vi "Overlay Line with Arrows Simple Modified.vi"(0 "Image In":T2, 1 "Group":string, 2 "Angle Coefficient":dbl, 5 "Line Coordinates":T1, 9 "Arrows":cluster{"Start point":bool, "End point":bool}, 11 "error in":errorcluster, 12 "Color":u32(colorbox)=16711680, 13 "Height Coefficient":dbl) -> (4 "Image Out":T2, 15 "error out":errorcluster)   [LabVIEW 2019]
uses:
  <vilib>/vision/Image Controls.llb/IMAQ Image.ctl
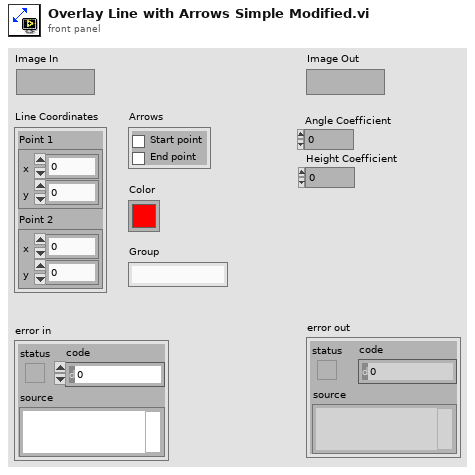
[diagram p1: front panel]
types:
  T1 = cluster{"Point 1":cluster{"x":dbl, "y":dbl}, "Point 2":cluster{"x":dbl, "y":dbl}}
  T2 = typedef "IMAQ Image.ctl" = refnum<image>
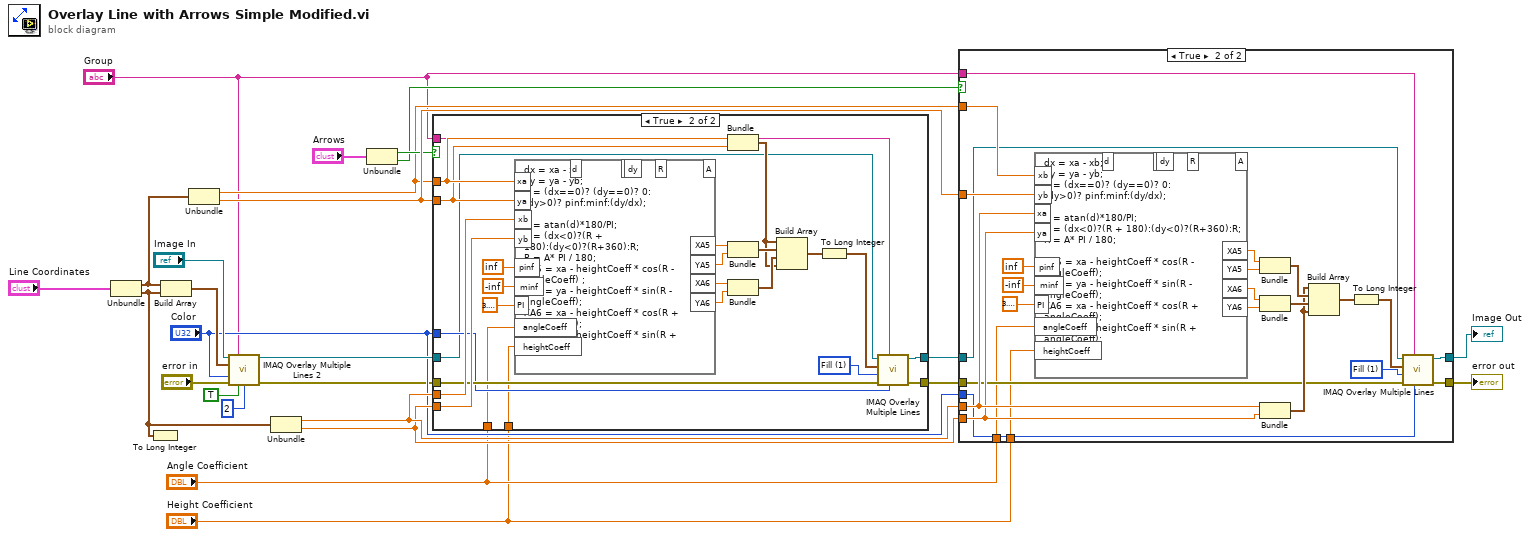
[diagram p0: block diagram]
diagram:
  n1 = Unbundle("Line Coordinates") -> ("Point 1"=w11:cluster{"x":dbl, "y":dbl}, "Point 2"=w10:cluster{"x":dbl, "y":dbl})
  n2 = To Long Integer(number=w10) -> ()  [unwired: 1 out]
  n3 = Build Array(w11, w10) -> (w9:cluster{"x":dbl, "y":dbl}[])
  n4 = Unbundle(w11) -> ("x"=w19:dbl, "y"=w24:dbl)
  n5 = call "IMAQ Overlay Multiple Lines 2"("Image"="Image In", "Group"="Group", "Line End Points"=w9, "Color"="Color", "error in (no error)"="error in", "Maintain Width?"=TRUE, "Width"=u32 2) -> ("Image Out"=w12:T2, "error out"=w6:errorcluster)  [unwired: 7 in]
  n6 = Unbundle(w10) -> ("x"=w23:dbl, "y"=w18:dbl)
  n7 = Unbundle("Arrows") -> ("Start point"=w22:bool, "End point"=w14:bool)
  n8 = case shown="True" w22 {
    tunnel: w19 -> [_ w41]
    tunnel: w24 -> [_ w40]
    tunnel: w23 -> [_ w42]
    tunnel: w18 -> [_ w39]
    tunnel: w12 -> [w27 w31]
    tunnel: [w27 w35] -> w20
    tunnel: "Color" -> [_ w32]
    tunnel: w6 -> [w26 w37]
    tunnel: [w26 w36] -> w17
    tunnel: "Group" -> [_ w30]
    tunnel: "Angle Coefficient" -> [_ w29]
    tunnel: "Height Coefficient" -> [_ w28]
    frame False {
    }
    frame True {
      w33 = u32 1 items=["Frame", "Fill"] ("Drawing Mode (Frame)")
      n9 = formula code="dx = xa - xb;\ndy = ya - yb;\nd = (dx==0)? (dy==0)? 0: \n(dy>0)? pinf:minf:(dy/dx);\n\nR = atan(d)*180/PI;\nA = (dx<0)?(R + 180):(dy<0)?(R+360):R;\nR = A* PI / 180;\nXA5 = xa - heightCoeff * cos(R - angleCoeff) ;\nYA5 = ya - heightCoeff * sin(R - angleCoeff);\nXA6 = xa - heightCoeff * cos(R + angleCoeff);\nYA6 = ya - heightCoeff * sin(R + angleCoeff);"("xa"=w41, "ya"=w40, "xb"=w42, "yb"=w39, "pinf"=inf, "minf"=-inf, "PI"=3.141592653589793, "angleCoeff"=w29, "heightCoeff"=w28) -> ("XA5"=w49:dbl, "YA5"=w48:dbl, "XA6"=w47:dbl, "YA6"=w46:dbl)  [unwired: 5 out]
      n10 = Bundle("x"=w41, "y"=w40) -> (w43:cluster{"x":dbl, "y":dbl})  [unwired: 1 out]
      n11 = Bundle("XA5"=w49, "YA5"=w48) -> (w45:cluster{"XA5":dbl, "YA5":dbl})  [unwired: 1 out]
      n12 = Bundle("XA6"=w47, "YA6"=w46) -> (w44:cluster{"XA6":dbl, "YA6":dbl})  [unwired: 1 out]
      n13 = Build Array(w43, w45, w44, w43) -> (w38:cluster{"x":dbl, "y":dbl}[])
      n14 = To Long Integer(number=w38) -> (32bit integer=w34:cluster{"x":i32, "y":i32}[])
      n15 = call "IMAQ Overlay Multiple Lines"("Color"=w32, "Group"=w30, "error in (no error)"=w37, "Drawing Mode (Frame)"=w33, "Line End Points"=w34, "Image"=w31) -> ("error out"=w36:errorcluster, "Image Out"=w35:T2)  [unwired: 4 out]
    }
  }
  n16 = case shown="True" w14 {
    tunnel: w19 -> [_ w76]
    tunnel: w24 -> [_ w75]
    tunnel: w23 -> [_ w74]
    tunnel: w18 -> [_ w73]
    tunnel: w20 -> [w54 w64]
    tunnel: [w54 w63] -> w21
    tunnel: "Color" -> [_ w59]
    tunnel: w17 -> [w53 w62]
    tunnel: [w53 w61] -> w16
    tunnel: "Group" -> [_ w57]
    tunnel: "Angle Coefficient" -> [_ w56]
    tunnel: "Height Coefficient" -> [_ w55]
    frame False {
    }
    frame True {
      w58 = u32 1 items=["Frame", "Fill"] ("Drawing Mode (Frame)")
      n17 = formula code="dx = xa - xb;\ndy = ya - yb;\nd = (dx==0)? (dy==0)? 0:\n(dy>0)? pinf:minf:(dy/dx);\n\nR = atan(d)*180/PI;\nA = (dx<0)?(R + 180):(dy<0)?(R+360):R;\nR = A* PI / 180;\n\nXA5 = xa - heightCoeff * cos(R - angleCoeff);\nYA5 = ya - heightCoeff * sin(R - angleCoeff);\nXA6 = xa - heightCoeff * cos(R + angleCoeff);\nYA6 = ya - heightCoeff * sin(R + angleCoeff);"("xb"=w76, "yb"=w75, "xa"=w74, "ya"=w73, "pinf"=inf, "minf"=-inf, "PI"=3.141592653589793, "angleCoeff"=w56, "heightCoeff"=w55) -> ("XA5"=w72:dbl, "YA5"=w71:dbl, "XA6"=w70:dbl, "YA6"=w69:dbl)  [unwired: 5 out]
      n18 = Bundle("XA5"=w72, "YA5"=w71) -> (w68:cluster{"XA5":dbl, "YA5":dbl})  [unwired: 1 out]
      n19 = Bundle("XA6"=w70, "YA6"=w69) -> (w67:cluster{"XA6":dbl, "YA6":dbl})  [unwired: 1 out]
      n20 = Bundle("x"=w74, "y"=w73) -> (w66:cluster{"x":dbl, "y":dbl})  [unwired: 1 out]
      n21 = Build Array(w66, w68, w67, w66) -> (w65:cluster{"x":dbl, "y":dbl}[])
      n22 = To Long Integer(number=w65) -> (32bit integer=w60:cluster{"x":i32, "y":i32}[])
      n23 = call "IMAQ Overlay Multiple Lines"("Color"=w59, "Group"=w57, "error in (no error)"=w62, "Drawing Mode (Frame)"=w58, "Line End Points"=w60, "Image"=w64) -> ("error out"=w61:errorcluster, "Image Out"=w63:T2)  [unwired: 4 out]
    }
  }
  "Image Out" <- w21
  "error out" <- w16
